vi "ReadMultipleSymbols_Sensata.vi"() -> ()   [LabVIEW 2020]
doc: "Read Multiple ADS Symbols using preconfigured blocks. The blocks are executed only once per VI run."
uses:
  <userlib>/Beckhoff-LabVIEW-Interface/_DependsOn/TypeDefs/Low-Levels/Symbol Interface Mode.ctl
  <userlib>/Beckhoff-LabVIEW-Interface/_DependsOn/With TypeResolving/Read Sync Single TypeResolved.vi
  <userlib>/Beckhoff-LabVIEW-Interface/_DependsOn/With TypeResolving/Read Async Single TypeResolved.vi
panel:
  out "element 3":string
  out "element 2":string
  out "element":string
  out "ReadGrpSymbols":string[](array[string])
  out "PortInfo":string
  out "error out":errorcluster
  in  "error in (no error)":errorcluster
  out "Data 3":variant
  out "Data 2":variant
  out "Data 1":variant
  out "Read Status? 3":bool
  out "Read Status? 2":bool
  out "Read Status?":bool
  in  "Symbol file path":path
  # "The example starts with retrieving read\nADS Symbols and selects the first symbol. The symbols can be selected:\n- Using Symbol file in symbol file path\n- Using Symbol Interface (UI), which is opened automatically if file path is empty.\n\nThe example reads, only once, the selected symbols in following order:\n- Symbol 1: synchronously therefore does wait for ADS response.\n- Symbol 2: asynchronously therefore does not wait for ADS response.\n- Symbol 3: same as symbol 1.\n\nThe example uses TypeResolvers to convert ADS row data to LabVIEW™ types.\n\nFor more information, please refer to block"
  # "Note: This example is only an illustration of all possible ways\nhow this Product can be used."
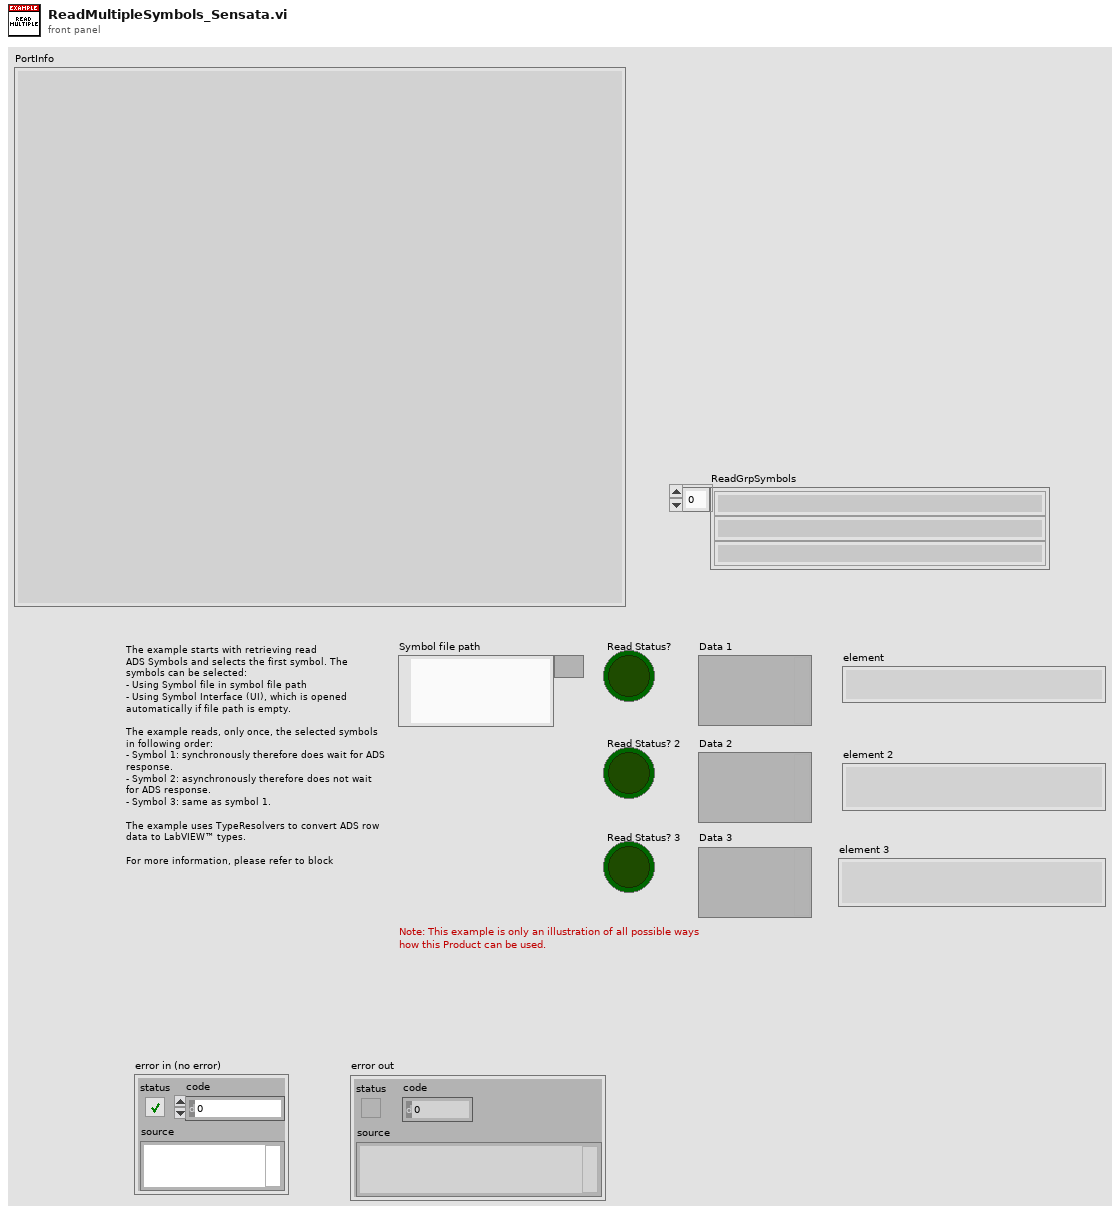
[diagram p1: front panel]
types:
  T1 = typedef "Symbol Interface Mode.ctl" = enum16{"Read Only", "Write Only", "Read & Write"}
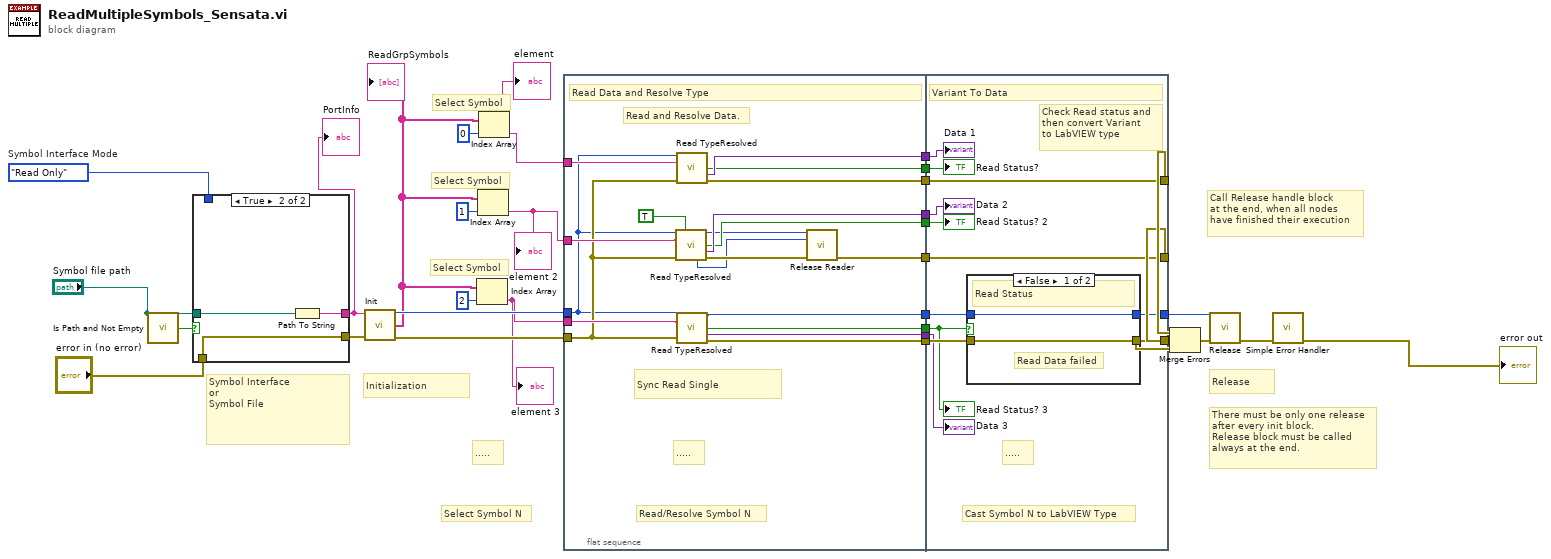
[diagram p0: block diagram]
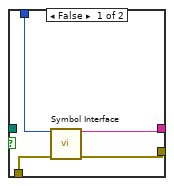
[diagram p2: hidden frame]
diagram:
  w5 = Symbol_Interface_Mode."Read Only"  # Symbol Interface Mode
  # "Symbol Interface\nor\nSymbol File"
  # "Call Release handle block\nat the end, when all nodes\nhave finished their execution"
  # "Select Symbol N"
  # "....."
  # "Select Symbol"
  # "Select Symbol"
  # "There must be only one release\nafter every init block.\nRelease block must be called\nalways at the end."
  # "Select Symbol"
  # "Initialization"
  # "Release"
  n1 = call <vilib>:"Is Path and Not Empty.vi"("path"="Symbol file path") -> ("Is Path and Not Empty?"=w8:bool)  [unwired: 4 in]
  n2 = case shown="True" w8 {
    tunnel: [w36 w39] -> w1
    tunnel: "Symbol file path" -> [_ w38]
    tunnel: [w35 w37] -> w7
    tunnel: w5 -> [w34 _]
    tunnel: "error in (no error)" -> [w33 w37]
    frame False {
      n3 = call <userlib>:"Symbol Interface.vi"("Symbol Interface Mode"=w34, "error in (no error)"=w33) -> ("PortInfo"=w36:string, "error out"=w35:errorcluster)  [unwired: 12 in]
    }
    frame True {
      n4 = Path To String(path=w38) -> (string=w39:string)
    }
  }
  "PortInfo" <- w1
  n5 = call <userlib>:"Init.vi"("XMLDescription"=w1, "error in (no error)"=w7) -> ("Handle"=w25:u32, "ReadGrpSymbols"=w12:string[], "error out"=w26:errorcluster)  [unwired: 9 in, 2 out]
  "ReadGrpSymbols" <- w12
  n6 = Index Array(array=w12, index=2) -> (element=w24:string)
  "element 3" <- w24
  n7 = Index Array(array=w12, index=1) -> (element=w28:string)
  "element 2" <- w28
  n8 = Index Array(array=w12, index=0) -> (element=w27:string)
  "element" <- w27
  n9 = flat-sequence {
    tunnel: w28 -> [w58]
    tunnel: w27 -> [w55]
    tunnel: w26 -> [w45]
    tunnel: w25 -> [w44]
    tunnel: w24 -> [w53]
    tunnel: [w42] -> w22
    tunnel: [w56] -> w21
    tunnel: [w54] -> w20
    tunnel: [w52] -> w19
    tunnel: [w51] -> w18
    tunnel: [w50] -> w17
    tunnel: [w49] -> w16
    tunnel: [w48] -> w15
    tunnel: [w47] -> w14
    tunnel: [w46] -> w13
    tunnel: [w65] -> w23
    tunnel: [w67] -> w9
    tunnel: [w70] -> w10
    tunnel: w22 -> [w70]
    tunnel: w21 -> [w69]
    tunnel: w20 -> [w66]
    tunnel: w19 -> [w68]
    tunnel: w18 -> [w61]
    tunnel: w17 -> [w60]
    tunnel: w16 -> [w59]
    tunnel: [w69] -> w11
    tunnel: w15 -> [w62]
    tunnel: w14 -> [w64]
    tunnel: w13 -> [w63]
    frame #0 {
      # "Read and Resolve Data."
      # "Read/Resolve Symbol N"
      # "....."
      # "Sync Read Single"
      # "Read Data and Resolve Type"
      n10 = call-poly <userlib>:"Read TypeResolved.vi"("Handle"=w44, "Wait?"=TRUE, "SymbolName"=w58, "error constant"=w45) -> ("Handle"=w41:u32, "Read Status?"=w46:bool, "RData"=w50:variant, "ReadHdl"=w40:u32, "error out"=w57:errorcluster)  [unwired: 6 in, 1 out]
      n11 = call-poly <userlib>:"Read TypeResolved.vi"("Handle"=w44, "SymbolName"=w55, "error constant"=w45) -> ("Read Status?"=w47:bool, "RData"=w51:variant, "error out"=w56:errorcluster)  [unwired: 9 in, 1 out]
      n12 = call-poly <userlib>:"Read TypeResolved.vi"("Handle"=w44, "SymbolName"=w53, "error constant"=w45) -> ("Handle"=w52:u32, "Read Status?"=w48:bool, "RData"=w49:variant, "error out"=w54:errorcluster)  [unwired: 9 in]
      n13 = call <userlib>:"Release Reader.vi"("Handle"=w41, "ReadHandle"=w40, "error in (no error)"=w57) -> ("error out"=w42:errorcluster)  [unwired: 11 in, 1 out]
    }
    frame #1 {
      # "Check Read status and\nthen convert Variant \nto LabVIEW type"
      # "Cast Symbol N to LabVIEW Type"
      # "....."
      # "Variant To Data"
      n14 = case shown="False" w62 {
        tunnel: w68 -> [w72 w73]
        tunnel: [w71 w74] -> w67
        tunnel: w66 -> [w71 w74]
        tunnel: [w72 w73] -> w65
        frame False {
          # "Read Data failed"
          # "Read Status"
        }
        frame True {
          # "User Code here"
          # "Variant to Data"
        }
      }
      "Read Status?" <- w64
      "Read Status? 2" <- w63
      "Read Status? 3" <- w62
      "Data 1" <- w61
      "Data 2" <- w60
      "Data 3" <- w59
    }
  }
  n15 = Merge Errors(w11, w10, w9) -> (w32:errorcluster)
  n16 = call <userlib>:"Release.vi"("Handle"=w23, "error in (no error)"=w32) -> ("error out"=w4:errorcluster)  [unwired: 13 in]
  n17 = call <vilib>:"Simple Error Handler.vi"("error in (no error)"=w4) -> ("error out"=→"error out":errorcluster)  [unwired: 4 in, 4 out]
